vi "DAQ_mx_queue.vi"() -> ()   [LabVIEW 2020]
uses:
  <vilib>/Utility/error.llb/DialogType.ctl
  <vilib>/Utility/sysdir.llb/System Directory Type.ctl
  <vilib>/DAQmx/read.llb/DAQmx Read (Analog 2D DBL NChan NSamp).vi
  <vilib>/DAQmx/create/channels.llb/DAQmx Create Channel (AI-Voltage-Basic).vi
  <vilib>/DAQmx/configure/timing.llb/DAQmx Timing (Sample Clock).vi
  <vilib>/DAQmx/configure/trigger.llb/DAQmx Start Trigger (None).vi
  <vilib>/DAQmx/miscellaneous.llb/DAQmx Fill In Error Info.vi
panel:
  in  "Save Button(顯性的)":bool
  in  "Save Button(隱性的)":bool
  out "Waveform Chart":dbl[][](graph)
  in  "stop":bool
  out "stop2":bool
  out "data":dbl[][](array[numeric])
  out "Waveform Chart 2":dbl[][](graph)
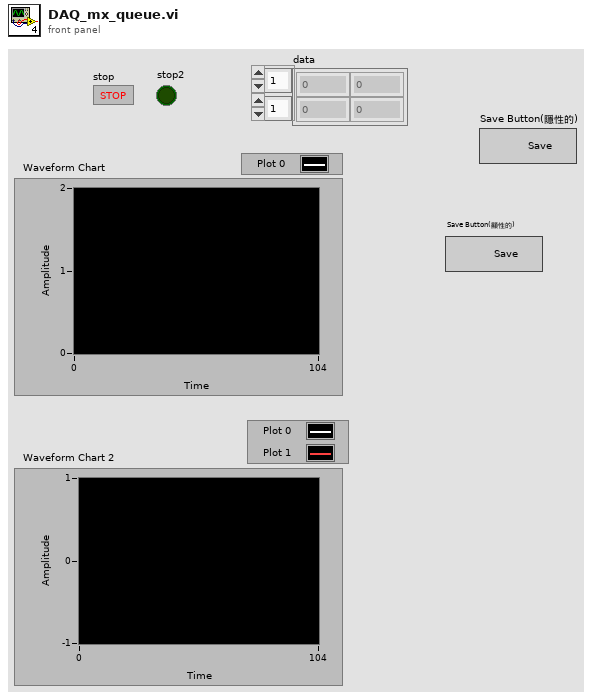
[diagram p1: front panel]
types:
  T1 = typedef "DialogType.ctl" = u16
  T2 = typedef "System Directory Type.ctl" = i32
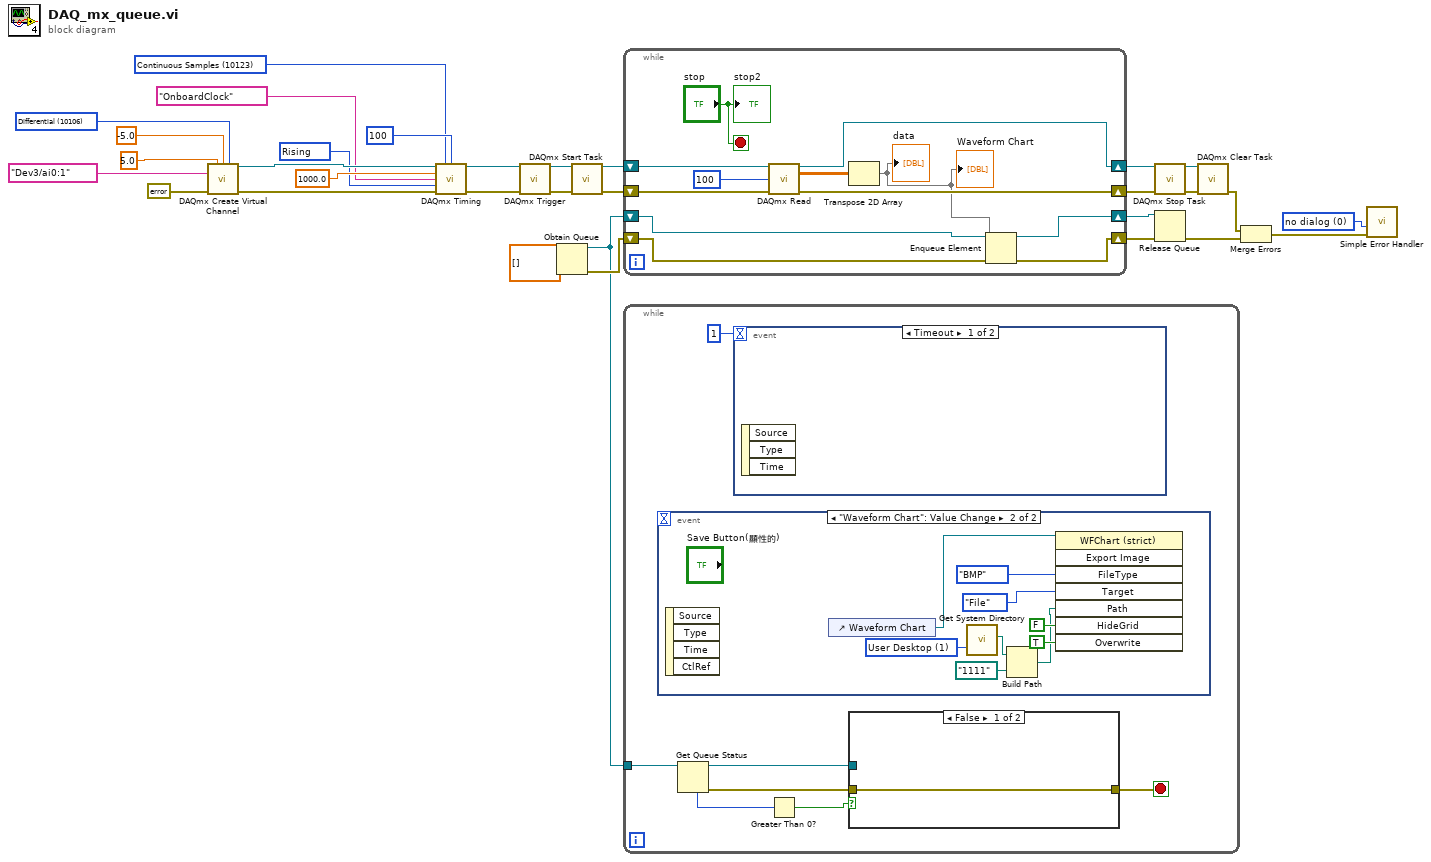
[diagram p0: block diagram]
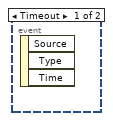
[diagram p2: hidden frame]
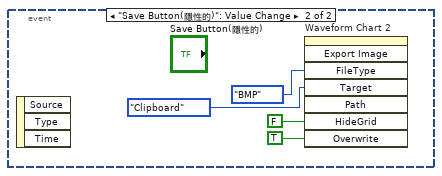
[diagram p3: hidden frame]
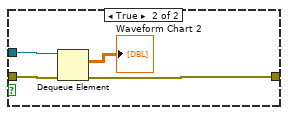
[diagram p4: hidden frame]
diagram:
  w9 = T1 0 items=["no dialog", "OK message", "continue or stop message", "OK message + warnings", "continue/stop + warnings"] ("type of dialog (OK msg:1)")
  w20 = 10280 items=["Rising"=10280, "Falling"=10171] ("active edge")
  w23 = 10123 items=["Finite Samples"=10178, "Continuous Samples"=10123, "Hardware Timed Single Point"=12522] ("sample mode")
  w31 = 10106 items=["Default"=-1, "RSE"=10083, "NRSE"=10078, "Differential"=10106, "Pseudodifferential"=12529] ("input terminal configuration")
  n1 = call-poly <vilib>:"DAQmx Create Virtual Channel.vi"("maximum value"=5.0, "minimum value"=-5.0, "input terminal configuration"=w31, "physical channels"=tag "Dev3/ai0:1", "error in"=errorcluster {"status"=FALSE, "code"=0, "source"=""}) -> ("task out"=w26:refnum<k21>, "error out"=w25:errorcluster)  [unwired: 9 in]
  n2 = call-poly <vilib>:"DAQmx Timing.vi"("task/channels in"=w26, "sample mode"=w23, "samples per channel"=100, "rate"=1000.0, "source"=tag "OnboardClock", "active edge"=w20, "error in"=w25) -> ("task out"=w19:refnum<k21>, "error out"=w18:errorcluster)  [unwired: 7 in]
  n3 = call-poly <vilib>:"DAQmx Trigger.vi"("task/channels in"=w19, "error in"=w18) -> ("task out"=w17:refnum<k21>, "error out"=w16:errorcluster)  [unwired: 12 in]
  n4 = Obtain Queue(element data type=dbl[][] []) -> (queue out=w1:refnum<queue>, error out=w7:errorcluster)  [unwired: 4 in, 1 out]
  n5 = call <vilib>:"DAQmx Start Task.vi"("task/channels in"=w17, "error in"=w16) -> ("task out"=w15:refnum<k21>, "error out"=w14:errorcluster)  [unwired: 12 in]
  n6 = while {
    shift-right: [w41] -> w13
    shift-left: w15 -> [w43]
    shift-right: [w40] -> w12
    shift-left: w14 -> [w42]
    shift-right: [w35] -> w6
    shift-left: w1 -> [w37]
    shift-right: [w34] -> w5
    shift-left: w7 -> [w36]
    stop <- "stop" stop-if-true
    n7 = call-poly <vilib>:"DAQmx Read.vi"("task/channels in"=w43, "number of samples per channel"=100 ("timeout"), "error in"=w42) -> ("task out"=w41:refnum<k21>, "data"=w33:dbl[][], "error out"=w40:errorcluster)  [unwired: 10 in]
    n8 = Transpose 2D Array(2D array=w33) -> (transposed array=w32:dbl[][])
    "Waveform Chart" <- w32
    "data" <- w32
    n9 = Enqueue Element(queue=w37, element=w32, error in (no error)=w36) -> (queue out=w35:refnum<queue>, error out=w34:errorcluster)  [unwired: 1 in, 1 out]
    "stop2" <- "stop"
  }
  n10 = while {
    tunnel: w1 -> [w49]
    stop <- w45 stop-if-true
    n11 = event shown="[1] \"Waveform Chart\": Value Change" {
      selector: _ -> [_ _]
      dyn-events: _ -> [_ _]
      timeout: _ -> [_ _]
      event Timeout {
        n12 = event-data() -> ()  [unwired: 1 in, 3 out]
      }
      event "Waveform Chart": Value Change {
        w54 = T2 1 items=["User Home"=0, "User Desktop"=1, "User Documents"=2, "User Application Data"=3, "User Preferences"=4, "User Temporary"=5, "Public Documents"=6, "Public Application Data"=7, "Public Preferences"=8, "Public Cache"=13, "System Core Libraries"=9, "System Installed Libraries"=10, "Application Files"=11, "Boot Volume Root"=12] ("system directory type")
        n13 = event-data() -> ()  [unwired: 1 in, 4 out]
        n14 = control-ref of="Waveform Chart"() -> (w59:refnum<vi>)
        n15 = call <vilib>:"Get System Directory.vi"("system directory type"=w54) -> ("system directory"=w53:path)  [unwired: 10 in]
        n16 = Build Path(base path=w53, name or relative path=path "1111") -> (appended path=w52:path)
        n17 = invoke class="WFChart (strict)" method="Export Image"(reference=w59, "FileType"=enum32{"BMP", "EPS", "EMF", "PICT"}."BMP" ("File Type"), "Target"=enum32{"File", "Clipboard"}."File", "Path"=w52, "HideGrid"=FALSE ("Hide Grid"), "Overwrite"=TRUE ("Always Overwrite")) -> ()  [unwired: 2 in, 8 out]
      }
    }
    n18 = Get Queue Status(queue=w49) -> (queue out=w47:refnum<queue>, error out=w46:errorcluster, # elements in queue=w50:i32)  [unwired: 2 in, 5 out]
    n19 = event shown="[0] Timeout" {
      selector: _ -> [_ _]
      dyn-events: _ -> [_ _]
      timeout: 1 -> [_ _]
      event Timeout {
        n20 = event-data() -> ()  [unwired: 1 in, 3 out]
      }
      event "Save Button(隱性的)": Value Change {
        n21 = event-data() -> ()  [unwired: 1 in, 3 out]
        n22 = invoke on="Waveform Chart 2" class="WFChart (strict)" method="Export Image"("FileType"=enum32{"BMP", "EPS", "EMF", "PICT"}."BMP" ("File Type"), "Target"=enum32{"File", "Clipboard"}."Clipboard", "HideGrid"=FALSE ("Hide Grid"), "Overwrite"=TRUE ("Always Overwrite")) -> ()  [unwired: 4 in, 8 out]
      }
    }
    n23 = Greater Than 0?(x=w50) -> (x > 0?=w48:bool)
    n24 = case shown="False" w48 {
      tunnel: w47 -> [_ w68]
      tunnel: w46 -> [w64 w67]
      tunnel: [w64 w65] -> w45
      frame False {
      }
      frame True {
        n25 = Dequeue Element(queue=w68, error in (no error)=w67) -> (element=→"Waveform Chart 2":dbl[][], error out=w65:errorcluster)  [unwired: 1 in, 2 out]
      }
    }
  }
  n26 = call <vilib>:"DAQmx Stop Task.vi"("task/channels in"=w13, "error in"=w12) -> ("task out"=w11:refnum<k21>, "error out"=w10:errorcluster)  [unwired: 12 in]
  n27 = Release Queue(queue=w6, error in (no error)=w5) -> (error out=w4:errorcluster)  [unwired: 1 in, 2 out]
  n28 = call <vilib>:"DAQmx Clear Task.vi"("task in"=w11, "error in"=w10) -> ("error out"=w3:errorcluster)  [unwired: 13 in]
  n29 = Merge Errors(w3, w4) -> (w2:errorcluster)
  n30 = call <vilib>:"Simple Error Handler.vi"("type of dialog (OK msg:1)"=w9, "error in (no error)"=w2) -> ()  [unwired: 3 in, 5 out]
